vi "Get All CD Parameters.vi"(8 "error in (no error)":errorcluster, 11 "Device Reference in":T18 format="%.0x") -> (0 "error out":errorcluster, 2 "VS References":T1={"Properties"={"Name"="", "CAN"={"Database File"=path "", "CAN Interface"=enum."CAN1", "Baud Rate"=0, "Diagnostic Protocol"=enum."GMLAN", "Transport Protocol"=enum."ISO TP - Normal Mode", "Transmit ID"=0, "Receive ID"=0, "Transmit Extension"=2, "Receive Extension"=1, "Receive UUDT ID"=0, "Enable Stream"=TRUE, "VW TP Channel ID"=0, "Security"={"Source DLL Path"=path "", "Security Level"=0, "Target DLL Path"=path ""}, "Fill Frame"=FALSE, "Fill Byte"=255, "Termination"=FALSE}, "FPGA Settings"={"RT Bitfile Path"=path "", "RIO Device"=0, "Enable"=FALSE}, "Reads"=[], "Frames Lookup"=variant(enum16{"GMLAN", "KWP-2000", "UDS"} enum."GMLAN"), "Writes"=[], "DPIDs"=[], "DPID Lookup"=variant(u32 0), "DTC descriptor"={"DTC Byte Length"=2, "Status Byte Length"=1, "Add Data Byte Length"=1, "Byte Order"=enum."Motorola"}}, "Refs"={"Read Data"=[], "Write Data"={"Refs"=[], "Values"=[]}, "Number of DTCs"=0, "DTCs"=[], "Status"=[], "Command Chanels"=[]}} {"Refs"."Command Chanels" format="%.0x"; "Refs"."Status" format="%.0x"; "Refs"."DTCs" format="%.0x"; "Refs"."Number of DTCs" format="%.0x"; "Refs"."Write Data"."Refs"."Data Reference" format="%.0x"; "Refs"."Read Data" format="%.0x"; "Properties"."Writes"."Signals"."Byte Order" items=["Little Endian", "Big Endian"]; "Properties"."Writes"."Signals"."Data Type" items=["Signed", "Unsigned", "IEEE Float"]; "Properties"."CAN"."Fill Byte" format="%.0x"; "Properties"."CAN"."VW TP Channel ID" format="%.0x"; "Properties"."CAN"."Receive UUDT ID" format="%.0x"; "Properties"."CAN"."Receive Extension" format="%.0x"; "Properties"."CAN"."Transmit Extension" format="%.0x"; "Properties"."CAN"."Receive ID" format="%.0x"; "Properties"."CAN"."Transmit ID" format="%.0x"; "Properties"."Reads"."Signals"."Byte Order" items=["Little Endian", "Big Endian"]; "Properties"."Reads"."Signals"."Data Type" items=["Signed", "Unsigned", "IEEE Float"]}, 3 "Device Reference out":T18 format="%.0x")   [LabVIEW 2015, in "Diagnostics Addon System Explorer.lvlib"]
uses:
  Diagnostics Addon System Explorer.lvlib
  <vilib>/NI Veristand/Custom Device API/Custom Device Item Ref.ctl
  Shared/Types/Compiled.Settings.ctl
  Shared/Types/Section Properties.ctl
  Shared/Types/CAN Configuration.ctl
  Shared/Types/CAN Interface.ctl
  Shared/Types/Diagnostic Protocols.ctl
  Shared/Types/Transport Protocols.ctl
  Shared/Types/Security.ctl
  Shared/Types/FPGA Bitfile Settings.ctl
  Shared/Types/Common Frame Parameters.ctl
  Shared/Types/MessageType Selector.ctl
  Shared/Types/Signal Parameters.ctl
  Shared/Types/DPID Parameters.ctl
  Shared/Types/DPID Periodic Rate.ctl
  <vilib>/Automotive Diagnostic Command Set/Diagnostic Protocols.llb/DTC Descriptor.ctl
  Shared/Types/Compiled.Refs.ctl
  <vilib>/NI Veristand/Custom Device API/Data Reference.ctl
  <vilib>/NI Veristand/Custom Device API/Block Data Reference.ctl
  <vilib>/NI Veristand/Custom Device API/Data Access Type.ctl
  Types/FG Action.ctl
  ID FG.vi
  Get Signals.vi
  Type FG.vi
  Create File Dependency.vi
  Shared/SubVIs/Calculate Frame Size.vi
  Signal Parameters FG.vi
  <vilib>/NI Veristand/Custom Device API/NI VeriStand - Get Item Property.vi
  <vilib>/NI Veristand/Custom Device API/Get Item Property (U32 Array).vi
  <vilib>/NI Veristand/Custom Device API/Get Item Property (U32).vi
  <vilib>/NI Veristand/Custom Device API/NI VeriStand - Set Item Property.vi
  <vilib>/NI Veristand/Custom Device API/Set Item Property (U32).vi
  Shared/SubVIs/GUID Lookup.vi
  <vilib>/NI Veristand/Custom Device API/Set Item Property (U32 Array).vi
  <vilib>/NI Veristand/Custom Device Tools/Custom Device Utility Library/NI VeriStand - Search for Item by GUID.vi
  <vilib>/NI Veristand/Custom Device API/Set Item Property (Boolean).vi
  <vilib>/NI Veristand/Custom Device API/NI VeriStand - Remove Item Property.vi
  <vilib>/NI Veristand/Custom Device API/Set Item Property (Dependent File).vi
  <vilib>/Utility/MD5Checksum.llb/MD5Checksum File.vi
  <vilib>/NI Veristand/Custom Device API/Set Item Property (Path).vi
  <vilib>/NI Veristand/Custom Device API/Get Item Property (Boolean).vi
  Get File Dependency Target Path.vi
  <vilib>/NI Veristand/Custom Device API/Get Item Property (Path).vi
  <vilib>/NI Veristand/Custom Device Tools/Custom Device Utility Library/NI VeriStand - Search for Item by Name.vi
  <vilib>/NI Veristand/Custom Device API/Get Item Property (I32).vi
  <vilib>/NI Veristand/Custom Device API/Set Item Property (I32).vi
  <vilib>/NI Veristand/Custom Device API/NI VeriStand - Get Channel Block Data References.vi
  <vilib>/NI Veristand/Custom Device API/NI VeriStand - Get Custom Device Channel Data.vi
  <vilib>/NI Veristand/Custom Device API/NI VeriStand - Get Item Description.vi
  <vilib>/NI Veristand/Custom Device API/Get Item Property (String).vi
  <vilib>/NI Veristand/Custom Device API/Get Item Property (Double).vi
  <vilib>/NI Veristand/Custom Device API/Set Item Property (String).vi
  <vilib>/NI Veristand/Custom Device API/Set Item Property (Double).vi
  <vilib>/NI Veristand/Custom Device Tools/Custom Device Utility Library/Custom Device Utility Library.lvlib
  Shared/Diagnostics Addon Shared.lvlib
  <vilib>/NI Veristand/Custom Device API/Custom Device API.lvlib
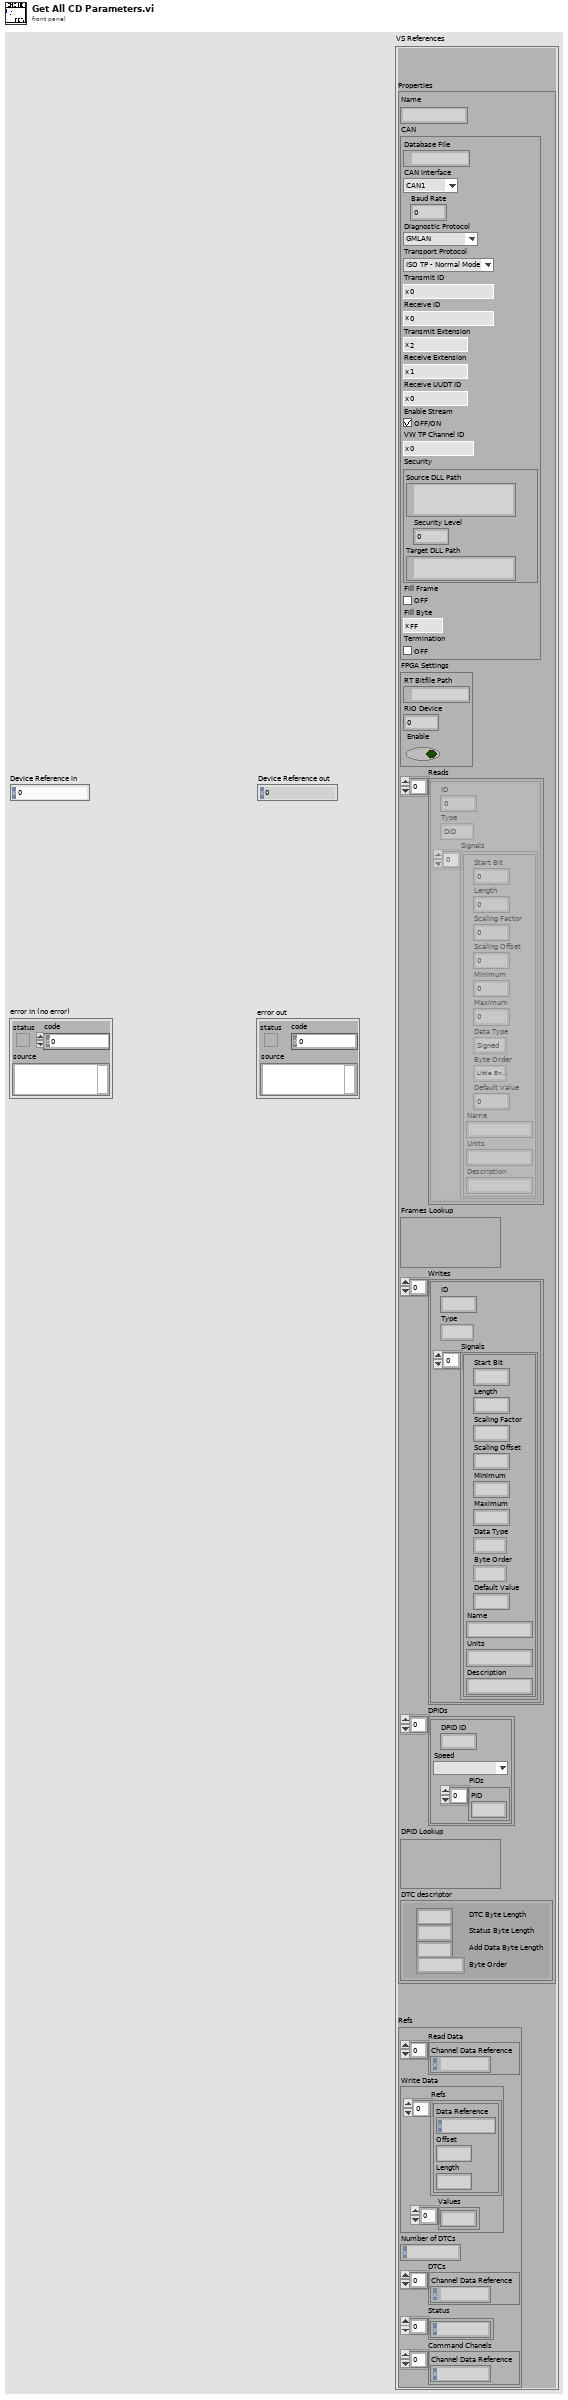
[diagram p1: front panel]
types:
  T1 = typedef "Diagnostics Addon Shared.lvlib/Compiled.Settings.ctl" = cluster{"Properties":T2, "Refs":T15}
  T2 = typedef "Diagnostics Addon Shared.lvlib/Section Properties.ctl" = cluster{"Name":string, "CAN":T3, "FPGA Settings":T8, "Reads":T9[], "Frames Lookup":variant, "Writes":T9[], "DPIDs":T12[], "DPID Lookup":variant, "DTC descriptor":T14}
  T3 = typedef "Diagnostics Addon Shared.lvlib/CAN Configuration.ctl" = cluster{"Database File":path, "CAN Interface":T4, "Baud Rate":u32, "Diagnostic Protocol":T5, "Transport Protocol":T6, "Transmit ID":u32, "Receive ID":u32, "Transmit Extension":u8, "Receive Extension":u8, "Receive UUDT ID":u32, "Enable Stream":bool, "VW TP Channel ID":u32, "Security":T7, "Fill Frame":bool, "Fill Byte":u8, "Termination":bool}
  T4 = typedef "Diagnostics Addon Shared.lvlib/CAN Interface.ctl" = enum16{"CAN0", "CAN1", "CAN2", "CAN3", "CAN4", "CAN5", "CAN6", "CAN7", "CAN8", "CAN9", "CAN10", "CAN11", "CAN12", "CAN13", "CAN14", "CAN15", "CAN16", "CAN17", "CAN18", "CAN19", "CAN20", "CAN21", "CAN22", "CAN23", "CAN24", "CAN25", "CAN26", "CAN27", "CAN28", "CAN29", "CAN30", "CAN31", "CAN32", "CAN33", "CAN34", "CAN35", "CAN36", "CAN37", "CAN38", "CAN39", "CAN40", "CAN41", "CAN42", "CAN43", "CAN44", "CAN45", "CAN46", "CAN47", "CAN48", "CAN49", "CAN50", "CAN51", "CAN52", "CAN53", "CAN54", "CAN55", "CAN56", "CAN57", "CAN58", "CAN59", "CAN60", "CAN61", "CAN62", "CAN63", "CAN 256 (Virtual)", "CAN 257 (Virtual)"}
  T5 = typedef "Diagnostics Addon Shared.lvlib/Diagnostic Protocols.ctl" = enum16{"GMLAN", "KWP-2000", "UDS"}
  T6 = typedef "Diagnostics Addon Shared.lvlib/Transport Protocols.ctl" = enum16{"ISO TP - Normal Mode", "ISO TP - Mixed Mode", "VW TP 2.0", "Diagnostics on IP"}
  T7 = typedef "Diagnostics Addon Shared.lvlib/Security.ctl" = cluster{"Source DLL Path":path, "Security Level":u8, "Target DLL Path":path}
  T8 = typedef "Diagnostics Addon Shared.lvlib/FPGA Bitfile Settings.ctl" = cluster{"RT Bitfile Path":path, "RIO Device":u16, "Enable":bool}
  T9 = typedef "Diagnostics Addon Shared.lvlib/Common Frame Parameters.ctl" = cluster{"ID":u32, "Type":T10, "Signals":T11[]}
  T10 = typedef "Diagnostics Addon Shared.lvlib/MessageType Selector.ctl" = enum16{"DID", "PID", "CPID", "Write Memory", "Read Memory", "DTC Control", "IO Cmd", "IO Resp", "Routine Start Cmd", "Routine Start Resp", "Routine Status Cmd", "Routine Status Resp", "Routine Stop Cmd", "Routine Stop Resp"}
  T11 = typedef "Diagnostics Addon Shared.lvlib/Signal Parameters.ctl" = cluster{"Start Bit":u8, "Length":u8, "Scaling Factor":dbl, "Scaling Offset":dbl, "Minimum":dbl, "Maximum":dbl, "Data Type":u32, "Byte Order":u32, "Default Value":dbl, "Name":string, "Units":string, "Description":string}
  T12 = typedef "Diagnostics Addon Shared.lvlib/DPID Parameters.ctl" = cluster{"DPID ID":u8, "Speed":T13, "PIDs":u16[]}
  T13 = typedef "Diagnostics Addon Shared.lvlib/DPID Periodic Rate.ctl" = enum16{"Slow", "Medium", "Fast"}
  T14 = typedef "Diagnostics Addon Shared.lvlib/DTC Descriptor.ctl" = cluster{"DTC Byte Length":i32, "Status Byte Length":i32, "Add Data Byte Length":i32, "Byte Order":enum16{"Motorola", "Intel"}}
  T15 = typedef "Diagnostics Addon Shared.lvlib/Compiled.Refs.ctl" = cluster{"Read Data":T16[], "Write Data":cluster{"Refs":T17[], "Values":dbl[]}, "Number of DTCs":T16, "DTCs":T16[], "Status":T16[], "Command Chanels":T16[]}
  T16 = typedef "Custom Device API.lvlib/Data Reference.ctl" = i32
  T17 = typedef "Custom Device API.lvlib/Block Data Reference.ctl" = cluster{"Data Reference":T16, "Offset":u64, "Length":u64}
  T18 = typedef "Custom Device API.lvlib/Custom Device Item Ref.ctl" = u64
  T19 = typedef "Diagnostics Addon System Explorer.lvlib/FG Action.ctl" = enum16{"Get", "Set"}
  T20 = typedef "Custom Device API.lvlib/Data Access Type.ctl" = enum16{"Read", "Write"}
  T21 = typedef "Diagnostics Addon System Explorer.lvlib/Frame Signal VS References.ctl" = cluster{"ID":u32, "Signal Refs":T18[]}
  T22 = typedef "Diagnostics Addon System Explorer.lvlib/Common IOs.ctl" = cluster{"Cmd":T9[], "Resp":T9[]}
  T23 = typedef "Diagnostics Addon System Explorer.lvlib/IO VS References.ctl" = cluster{"Cmd":T21[], "Resp":T21[]}
  T24 = typedef "Diagnostics Addon System Explorer.lvlib/Common Routines.ctl" = cluster{"Start.Cmd":T9[], "Start.Resp":T9[], "Request.Cmd":T9[], "Request.Resp":T9[], "Stop.Cmd":T9[], "Stop.Resp":T9[]}
  T25 = typedef "Diagnostics Addon System Explorer.lvlib/Routine VS References.ctl" = cluster{"Start.Cmd":T21[], "Start.Resp":T21[], "Status.Cmd":T21[], "Status.Resp":T21[], "Stop.Cmd":T21[], "Stop.Resp":T21[]}
  T26 = typedef "Custom Device API.lvlib/Custom Device Item Info.ctl" = cluster{"Name":string, "Is Channel":bool, "GUID":string, "Is Waveform":bool}
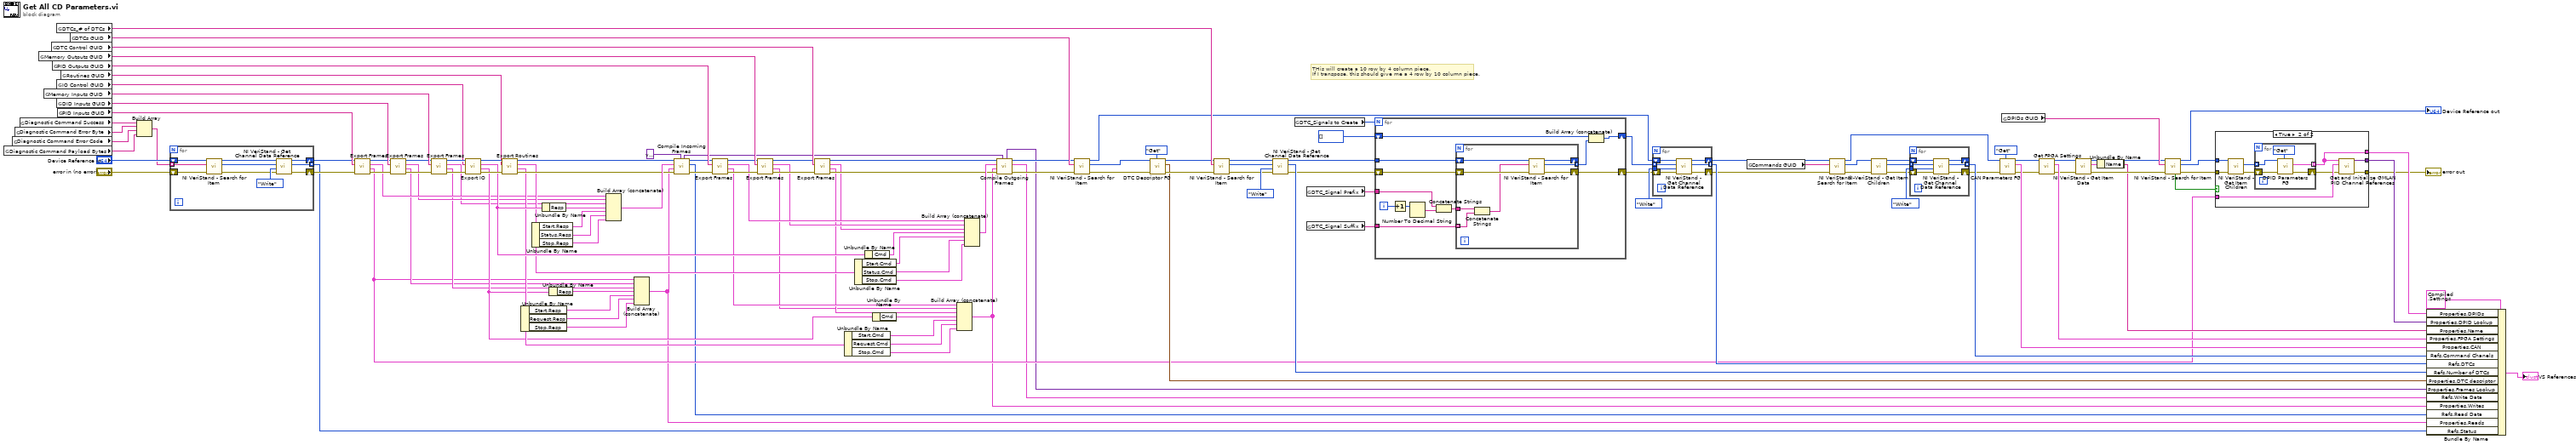
[diagram p0: block diagram]
diagram:
  # "THis will create a 10 row by 4 column piece.\nIf I transpose, this should give me a 4 row by 10 column piece."
  n1 = global read "GUID Lookup.vi" "Diagnostic Command Payload Bytes"() -> (w4:string)
  n2 = global read "GUID Lookup.vi" "Diagnostic Command Error Code"() -> (w3:string)
  n3 = global read "GUID Lookup.vi" "Diagnostic Command Error Byte"() -> (w5:string)
  n4 = global read "GUID Lookup.vi" "Diagnostic Command Success"() -> (w6:string)
  n5 = global read "GUID Lookup.vi" "Memory Outputs GUID"() -> (w79:string)
  n6 = global read "GUID Lookup.vi" "Memory Inputs GUID"() -> (w78:string)
  n7 = global read "GUID Lookup.vi" "DTC Control GUID"() -> (w62:string)
  n8 = global read "GUID Lookup.vi" "PID Outputs GUID"() -> (w124:string)
  n9 = global read "GUID Lookup.vi" "DTCs_# of DTCs"() -> (w135:string)
  n10 = global read "GUID Lookup.vi" "IO Control GUID"() -> (w47:string)
  n11 = global read "GUID Lookup.vi" "DID Inputs GUID"() -> (w125:string)
  n12 = global read "GUID Lookup.vi" "PID Inputs GUID"() -> (w123:string)
  n13 = global read "GUID Lookup.vi" "Routines GUID"() -> (w46:string)
  n14 = global read "GUID Lookup.vi" "DTCs GUID"() -> (w136:string)
  n15 = Build Array(w6, w5, w3, w4) -> (w2:string[])
  n16 = for {
    tunnel: w2 -> [w144] mode=indexing
    tunnel: [w139] -> w1 mode=indexing
    shift-right: [w138] -> w8
    shift-left: "error in (no error)" -> [w146]
    shift-right: [w137] -> w7
    shift-left: "Device Reference in" -> [w145]
    n17 = call-poly <vilib>:"NI VeriStand - Search for Item.vi"("error in"=w146, "Item Name"=w144, "Section Ref in"=w145) -> ("error out"=w142:errorcluster, "Item Ref"=w140:T18, "Section Ref out"=w141:T18)  [unwired: 5 in, 1 out]
    n18 = call <vilib>:"NI VeriStand - Get Channel Data Reference.vi"("error in (no error)"=w142, "Access"=Data_Access_Type."Write", "Channel Ref in"=w140, "Device Ref in"=w141) -> ("error out"=w138:errorcluster, "Channel Data Reference"=w139:T16, "Device Ref out"=w137:T18)  [unwired: 5 in]
  }
  n19 = call "Export Frames.vi"("error in (no error)"=w8, "GUID"=w123, "Section Ref in"=w7) -> ("error out"=w65:errorcluster, "Frame Settings Array"=w30:T9[], "Frame Refs"=w43:T21[], "Section Ref out"=w77:T18)  [unwired: 5 in]
  n20 = call "Export Frames.vi"("error in (no error)"=w65, "GUID"=w125, "Section Ref in"=w77) -> ("error out"=w66:errorcluster, "Frame Settings Array"=w31:T9[], "Frame Refs"=w42:T21[], "Section Ref out"=w76:T18)  [unwired: 5 in]
  n21 = call "Export Frames.vi"("error in (no error)"=w66, "GUID"=w78, "Section Ref in"=w76) -> ("error out"=w67:errorcluster, "Frame Settings Array"=w32:T9[], "Frame Refs"=w41:T21[], "Section Ref out"=w75:T18)  [unwired: 5 in]
  n22 = call "Export IO.vi"("error in (no error)"=w67, "GUID"=w47, "Section Ref in"=w75) -> ("error out"=w68:errorcluster, 1:"IO"=w44:T22, 2:"IO"=w57:T23, "Section Ref out"=w74:T18)  [unwired: 5 in]
  n23 = call "Export Routines.vi"("error in (no error)"=w68, "GUID"=w46, "Section Ref in"=w74) -> ("error out"=w71:errorcluster, "Routines"=w45:T24, "Routine Refs"=w56:T25, "Section Ref out"=w72:T18)  [unwired: 5 in]
  n24 = Unbundle By Name(w45) -> ("Start.Resp"=w36:T9[], "Request.Resp"=w35:T9[], "Stop.Resp"=w34:T9[])
  n25 = Unbundle By Name(w56) -> ("Start.Resp"=w39:T21[], "Status.Resp"=w38:T21[], "Stop.Resp"=w37:T21[])
  n26 = Unbundle By Name(w57) -> ("Resp"=w40:T21[])
  n27 = Unbundle By Name(w44) -> ("Resp"=w33:T9[])
  n28 = Build Array (concatenate)(w43, w42, w41, w40, w39, w38, w37) -> (w73:T21[])
  n29 = Build Array (concatenate)(w30, w31, w32, w33, w36, w35, w34) -> (w14:T9[])
  n30 = call "Compile Incoming Frames.vi"("Lookups in"=variant, "error in (no error)"=w71, "Frame Settings Array"=w14, "Refs"=w73, "Item Ref in"=w72) -> ("error out"=w70:errorcluster, "Refs"=w11:T16[], "Item Ref out"=w69:T18, "Lookups"=w10:variant)  [unwired: 3 in]
  n31 = call "Export Frames.vi"("error in (no error)"=w70, "GUID"=w124, "Section Ref in"=w69) -> ("error out"=w58:errorcluster, "Frame Settings Array"=w22:T9[], "Frame Refs"=w29:T21[], "Section Ref out"=w61:T18)  [unwired: 5 in]
  n32 = call "Export Frames.vi"("error in (no error)"=w58, "GUID"=w79, "Section Ref in"=w61) -> ("error out"=w59:errorcluster, "Frame Settings Array"=w16:T9[], "Frame Refs"=w28:T21[], "Section Ref out"=w60:T18)  [unwired: 5 in]
  n33 = call "Export Frames.vi"("error in (no error)"=w59, "GUID"=w62, "Section Ref in"=w60) -> ("error out"=w54:errorcluster, "Frame Settings Array"=w17:T9[], "Frame Refs"=w27:T21[], "Section Ref out"=w53:T18)  [unwired: 5 in]
  n34 = Unbundle By Name(w45) -> ("Start.Cmd"=w19:T9[], "Request.Cmd"=w20:T9[], "Stop.Cmd"=w21:T9[])
  n35 = Unbundle By Name(w56) -> ("Start.Cmd"=w25:T21[], "Status.Cmd"=w24:T21[], "Stop.Cmd"=w23:T21[])
  n36 = Unbundle By Name(w57) -> ("Cmd"=w26:T21[])
  n37 = Unbundle By Name(w44) -> ("Cmd"=w18:T9[])
  n38 = Build Array (concatenate)(w22, w16, w17, w18, w19, w20, w21) -> (w15:T9[])
  n39 = Build Array (concatenate)(w29, w28, w27, w26, w25, w24, w23) -> (w55:T21[])
  n40 = call "Compile Outgoing Frames.vi"("Lookup In"=w10, "error in (no error)"=w54, "Frame Settings Array"=w15, "Refs"=w55, "Item Ref in"=w53) -> ("error out"=w52:errorcluster, "Refs"=w13:cluster{"Refs":T17[], "Values":dbl[]}, "Item Ref out"=w51:T18, "Lookup"=w12:variant)  [unwired: 3 in]
  n41 = call-poly <vilib>:"NI VeriStand - Search for Item.vi"("error in"=w52, "Item GUID"=w136, "Section Ref in"=w51) -> ("error out"=w98:errorcluster, "Item Ref"=w96:T18, "Section Ref out"=w114:T18)  [unwired: 5 in, 1 out]
  n42 = call "DTC Descriptor FG.vi"("Action"=FG_Action."Get", "error in (no error)"=w98, "Device Item Ref in"=w96) -> ("error out"=w97:errorcluster, "DTC descriptor"=w94:T14, "Device Item Ref out"=w95:T18)  [unwired: 6 in]
  n43 = call-poly <vilib>:"NI VeriStand - Search for Item.vi"("error in"=w97, "Item Name"=w135, "Section Ref in"=w95) -> ("error out"=w110:errorcluster, "Item Ref"=w113:T18, "Section Ref out"=w108:T18)  [unwired: 5 in, 1 out]
  n44 = call <vilib>:"NI VeriStand - Get Channel Data Reference.vi"("error in (no error)"=w110, "Access"=Data_Access_Type."Write", "Channel Ref in"=w113, "Device Ref in"=w108) -> ("error out"=w109:errorcluster, "Channel Data Reference"=w112:T16, "Device Ref out"=w107:T18)  [unwired: 5 in]
  n45 = global read "GUID Lookup.vi" "DTC_Signals to Create"() -> (w132:i32)
  n46 = global read "GUID Lookup.vi" "DTC_Signal Prefix"() -> (w134:string)
  n47 = global read "GUID Lookup.vi" "DTC_Signal Suffix"() -> (w133:string[])
  n48 = for {
    N: w132 -> [_]
    tunnel: w107 -> [w158]
    shift-right: [w156] -> w116
    shift-left: w109 -> [w157]
    tunnel: w133 -> [w151]
    tunnel: w134 -> [w150]
    shift-right: [w147] -> w115
    shift-left: T18[] [] -> [w149]
    i -> [w153]
    n49 = Increment(x=w153) -> (x+1=w155:i32)
    n50 = Number To Decimal String(number=w155) -> (decimal integer string=w154:string)  [unwired: 1 in]
    n51 = Concatenate Strings(w150, w154) -> (w152:string)
    n52 = for {
      shift-right: [w165] -> _
      shift-left: w158 -> [w166]
      shift-right: [w163] -> w156
      shift-left: w157 -> [w164]
      tunnel: w151 -> [w162] mode=indexing
      tunnel: w152 -> [w161]
      tunnel: [w159] -> w148 mode=indexing
      n53 = Concatenate Strings(w161, w162) -> (w160:string)
      n54 = call-poly <vilib>:"NI VeriStand - Search for Item.vi"("error in"=w164, "Item Name"=w160, "Section Ref in"=w166) -> ("error out"=w163:errorcluster, "Item Ref"=w159:T18, "Section Ref out"=w165:T18)  [unwired: 5 in, 1 out]
    }
    n55 = Build Array (concatenate)(w149, w148) -> (w147:T18[])
  }
  n56 = for {
    tunnel: w115 -> [w169] mode=indexing
    tunnel: Data_Access_Type."Write" ("Access") -> [w168]
    shift-right: [w171] -> w64
    shift-left: w116 -> [w172]
    shift-right: [w173] -> w63
    shift-left: w114 -> [w170]
    tunnel: [w167] -> w88 mode=indexing
    n57 = call <vilib>:"NI VeriStand - Get Channel Data Reference.vi"("error in (no error)"=w172, "Access"=w168, "Channel Ref in"=w169, "Device Ref in"=w170) -> ("error out"=w171:errorcluster, "Channel Data Reference"=w167:T16, "Device Ref out"=w173:T18)  [unwired: 5 in]
  }
  n58 = global read "GUID Lookup.vi" "Commands GUID"() -> (w128:string)
  n59 = call-poly <vilib>:"NI VeriStand - Search for Item.vi"("error in"=w64, "Item GUID"=w128, "Section Ref in"=w63) -> ("error out"=w127:errorcluster, "Item Ref"=w126:T18, "Section Ref out"=w100:T18)  [unwired: 5 in, 1 out]
  n60 = call <vilib>:"NI VeriStand - Get Item Children.vi"("error in (no error)"=w127, "Item Ref in"=w126) -> ("error out"=w121:errorcluster, "Child Refs"=w119:T18[], "Item Ref out"=w120:T18)  [unwired: 6 in, 1 out]
  n61 = for {
    tunnel: w119 -> [w176] mode=indexing
    tunnel: Data_Access_Type."Write" ("Access") -> [w175]
    shift-right: [w178] -> w101
    shift-left: w121 -> [w179]
    shift-right: [w180] -> _
    shift-left: w120 -> [w177]
    tunnel: [w174] -> w118 mode=indexing
    n62 = call <vilib>:"NI VeriStand - Get Channel Data Reference.vi"("error in (no error)"=w179, "Access"=w175, "Channel Ref in"=w176, "Device Ref in"=w177) -> ("error out"=w178:errorcluster, "Channel Data Reference"=w174:T16, "Device Ref out"=w180:T18)  [unwired: 5 in]
  }
  n63 = call "CAN Parameters FG.vi"("Action"=FG_Action."Get", "error in (no error)"=w101, "Device Item Ref in"=w100) -> ("error out"=w91:errorcluster, "Diagnostics Basic Configuraiton"=w92:T3, "Device Item Ref out"=w90:T18)  [unwired: 6 in]
  n64 = global read "GUID Lookup.vi" "DPIDs GUID"() -> (w105:string)
  n65 = call "Get FPGA Settings.vi"("error in (no error)"=w91, "Item Ref in"=w90) -> ("error out"=w85:errorcluster, "FPGA Bitfile Settings"=w89:T8, "Item Ref out"=w83:T18)  [unwired: 7 in]
  n66 = call <vilib>:"NI VeriStand - Get Item Data.vi"("error in (no error)"=w85, "Item Ref in"=w83) -> ("error out"=w84:errorcluster, "Item Info"=w86:T26, "Item Ref out"=w82:T18)  [unwired: 6 in, 1 out]
  n67 = Unbundle By Name(w86) -> ("Name"=w81:string)
  n68 = call-poly <vilib>:"NI VeriStand - Search for Item.vi"("error in"=w84, "Item GUID"=w105, "Section Ref in"=w82) -> ("error out"=w106:errorcluster, "Item Ref"=w104:T18, "Section Ref out"=→"Device Reference out":T18, "Found"=w102:bool)  [unwired: 5 in]
  n69 = case shown="True" w102 {
    tunnel: w106 -> [w181 w190]
    tunnel: w104 -> [_ w187]
    tunnel: [w181 w184] -> w49
    tunnel: [_ w182] -> w93
    tunnel: w30 -> [_ w186]
    tunnel: [_ w183] -> w80
    frame False {
    }
    frame True {
      n70 = call <vilib>:"NI VeriStand - Get Item Children.vi"("error in (no error)"=w190, "Item Ref in"=w187) -> ("error out"=w189:errorcluster, "Child Refs"=w188:T18[])  [unwired: 6 in, 2 out]
      n71 = for {
        tunnel: w188 -> [w194] mode=indexing
        tunnel: [w193] -> w182 mode=indexing
        shift-right: [w192] -> w185
        shift-left: w189 -> [w195]
        n72 = call "DPID Parameters FG.vi"("Action"=FG_Action."Get", "error in (no error)"=w195, "Device Item Ref in"=w194) -> ("error out"=w192:errorcluster, "DPID"=w193:T12)  [unwired: 6 in, 1 out]
      }
      n73 = call "Get and Initialize GMLAN PID Channel References.vi"("error in (no error)"=w185, "PIDs"=w186, "DPIDs"=w182) -> ("error out"=w184:errorcluster, "Lookup Table"=w183:variant)  [unwired: 7 in]
    }
  }
  "error out" <- w49
  n74 = Bundle By Name(cluster=T1 {"Properties"={"Name"="", "CAN"={"Database File"=path "", "CAN Interface"=enum."CAN1", "Baud Rate"=0, "Diagnostic Protocol"=enum."GMLAN", "Transport Protocol"=enum."ISO TP - Normal Mode", "Transmit ID"=0, "Receive ID"=0, "Transmit Extension"=2, "Receive Extension"=1, "Receive UUDT ID"=0, "Enable Stream"=TRUE, "VW TP Channel ID"=0, "Security"={"Source DLL Path"=path "", "Security Level"=0, "Target DLL Path"=path ""}, "Fill Frame"=FALSE, "Fill Byte"=255, "Termination"=FALSE}, "FPGA Settings"={"RT Bitfile Path"=path "", "RIO Device"=0, "Enable"=FALSE}, "Reads"=[], "Frames Lookup"=variant(enum16{"GMLAN", "KWP-2000", "UDS"} enum."GMLAN"), "Writes"=[], "DPIDs"=[], "DPID Lookup"=variant(u32 0), "DTC descriptor"={"DTC Byte Length"=2, "Status Byte Length"=1, "Add Data Byte Length"=1, "Byte Order"=enum."Motorola"}}, "Refs"={"Read Data"=[], "Write Data"={"Refs"=[], "Values"=[]}, "Number of DTCs"=0, "DTCs"=[], "Status"=[], "Command Chanels"=[]}} ("VS References"), "Properties.DPIDs"=w93, "Properties.DPID Lookup"=w80, "Properties.Name"=w81, "Properties.FPGA Settings"=w89, "Properties.CAN"=w92, "Refs.Command Chanels"=w118, "Refs.DTCs"=w88, "Refs.Number of DTCs"=w112, "Properties.DTC descriptor"=w94, "Properties.Frames Lookup"=w12, "Refs.Write Data"=w13, "Properties.Writes"=w15, "Refs.Read Data"=w11, "Properties.Reads"=w14, "Refs.Status"=w1) -> (→"VS References":T1)
